vi "Calibrate Timeout 2 Ticks (uSMC).vi"(1 "Timeout (ms)":u16) -> (0 "Timeout (Ticks)":u16)   [LabVIEW 2010, in "SignalWriterMH110203USBStepperMotor.lvclass"]
uses:
  SignalWriterMH110203USBStepperMotor.lvclass
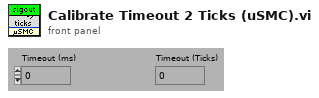
[diagram p1: front panel]
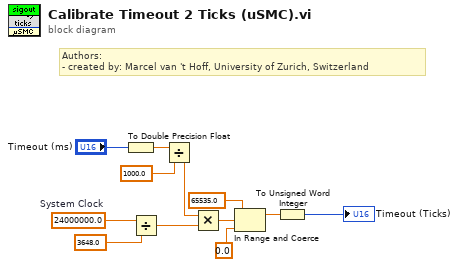
[diagram p0: block diagram]
diagram:
  w12 = 24000000.0  # System Clock
  # "Authors: \n- created by: Marcel van 't Hoff, University of Zurich, Switzerland"
  n1 = To Double Precision Float(number="Timeout (ms)") -> (double precision float=w3:dbl)
  n2 = Divide(x=w12, y=3648.0) -> (x/y=w4:dbl)
  n3 = Divide(x=w3, y=1000.0) -> (x/y=w2:dbl)
  n4 = Multiply(x=w2, y=w4) -> (x*y=w8:dbl)
  n5 = In Range and Coerce(upper limit=65535.0, x=w8, lower limit=0.0) -> (coerced(x)=w7:dbl)  [unwired: 1 out]
  n6 = To Unsigned Word Integer(number=w7) -> (unsigned 16bit integer=→"Timeout (Ticks)":u16)
